vi "sub_setAlternateCellValue.vi"(9 "invalid guess":T1, 11 "solver (in) array":cluster{"solved":bool, "values":string[]}[][](array[cluster])) -> (3 "solver (out)":cluster{"solved":bool, "values":string[]}[][](array[cluster]))   [LabVIEW 2018]
uses:
  guess.ctl
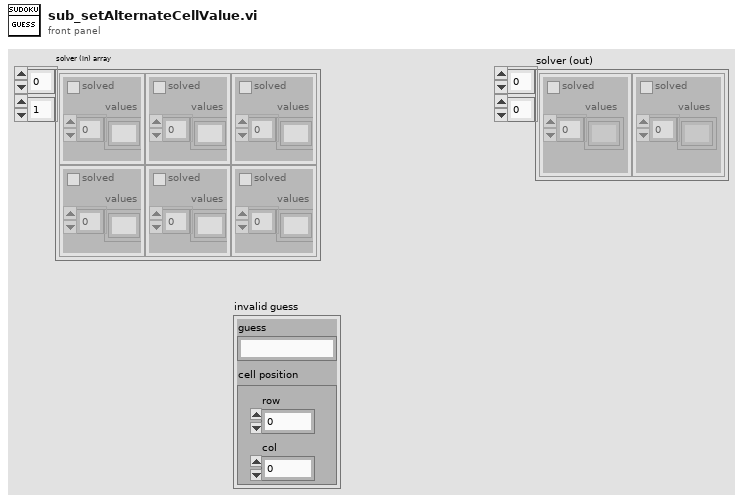
[diagram p1: front panel]
types:
  T1 = typedef "guess.ctl" = cluster{"cell position":cluster{"row":i32, "col":i32}, "guess":string}
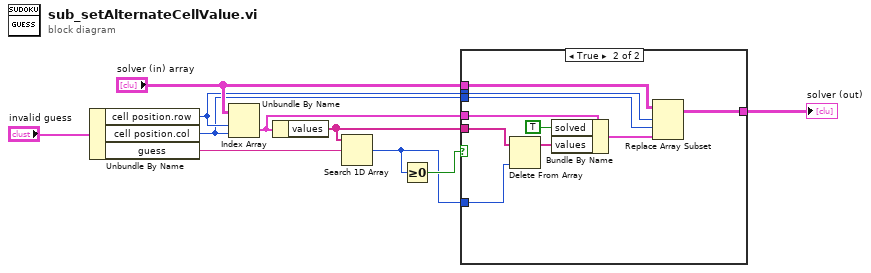
[diagram p0: block diagram]
diagram:
  n1 = Unbundle By Name("invalid guess") -> ("cell position.row"=w8:i32, "cell position.col"=w7:i32, "guess"=w6:string)
  n2 = Index Array(array="solver (in) array", index (row)=w8, index (col)=w7) -> (element=w3:cluster{"solved":bool, "values":string[]})
  n3 = Unbundle By Name(w3) -> ("values"=w4:string[])
  n4 = Search 1D Array(1D array=w4, element=w6) -> (index of element=w1:i32)  [unwired: 1 in]
  n5 = Greater Or Equal To 0?(x=w1) -> (x >= 0?=w2:bool)
  n6 = case shown="True" w2 {
    tunnel: "solver (in) array" -> [w11 w21]
    tunnel: w8 -> [_ w20]
    tunnel: w7 -> [_ w19]
    tunnel: [w11 w18] -> w5
    tunnel: w4 -> [_ w17]
    tunnel: w3 -> [_ w16]
    tunnel: w1 -> [_ w12]
    frame False {
    }
    frame True {
      n7 = Delete From Array(array=w17, index=w12) -> (array with subset deleted=w14:string[])  [unwired: 1 in, 1 out]
      n8 = Bundle By Name(cluster=w16, "solved"=TRUE, "values"=w14) -> (w13:cluster{"solved":bool, "values":string[]})
      n9 = Replace Array Subset(array=w21, new element=w13, index (row)=w20, index (col)=w19) -> (w18:cluster{"solved":bool, "values":string[]}[][])
    }
  }
  "solver (out)" <- w5
